vi "Start Process.vi"(0 "Stop / Start Reactor X":refnum<vi>, 1 "System Idle Pressure X":refnum<vi>, 2 "Reactor Number":i32, 3 "Logging Data X":refnum<vi>, 4 "Save File Connection X":refnum<vi>, 5 "Save File JSON Connection X":refnum<vi>, 6 "Header Connection txt Array":refnum<vi>, 7 "Queue Reactor X":refnum<vi>, 8 "Start Time Reactor X":refnum<vi>, 9 "Queue System":refnum<vi>, 10 "Username X":refnum<vi>, 11 "Current Locks":refnum<vi>, 12 "Experimental Details X":refnum<vi>, 13 "System JSON Queue":refnum<vi>, 14 "ALD Sequence for Reactor X":refnum<vi>, 15 "Stop Program":refnum<vi>, 16 "Number of Shared Lines":i32, 17 "Lock Reentrance Rate":u32, 18 "GUID X":refnum<vi>, 19 "Reactor Name":string) -> ()   [LabVIEW 2021]
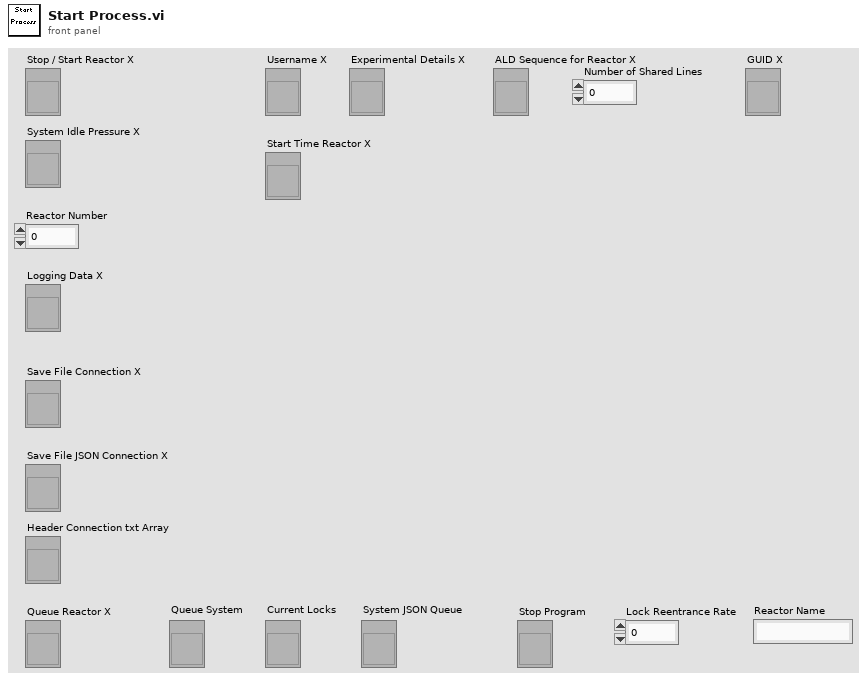
[diagram p1: front panel]
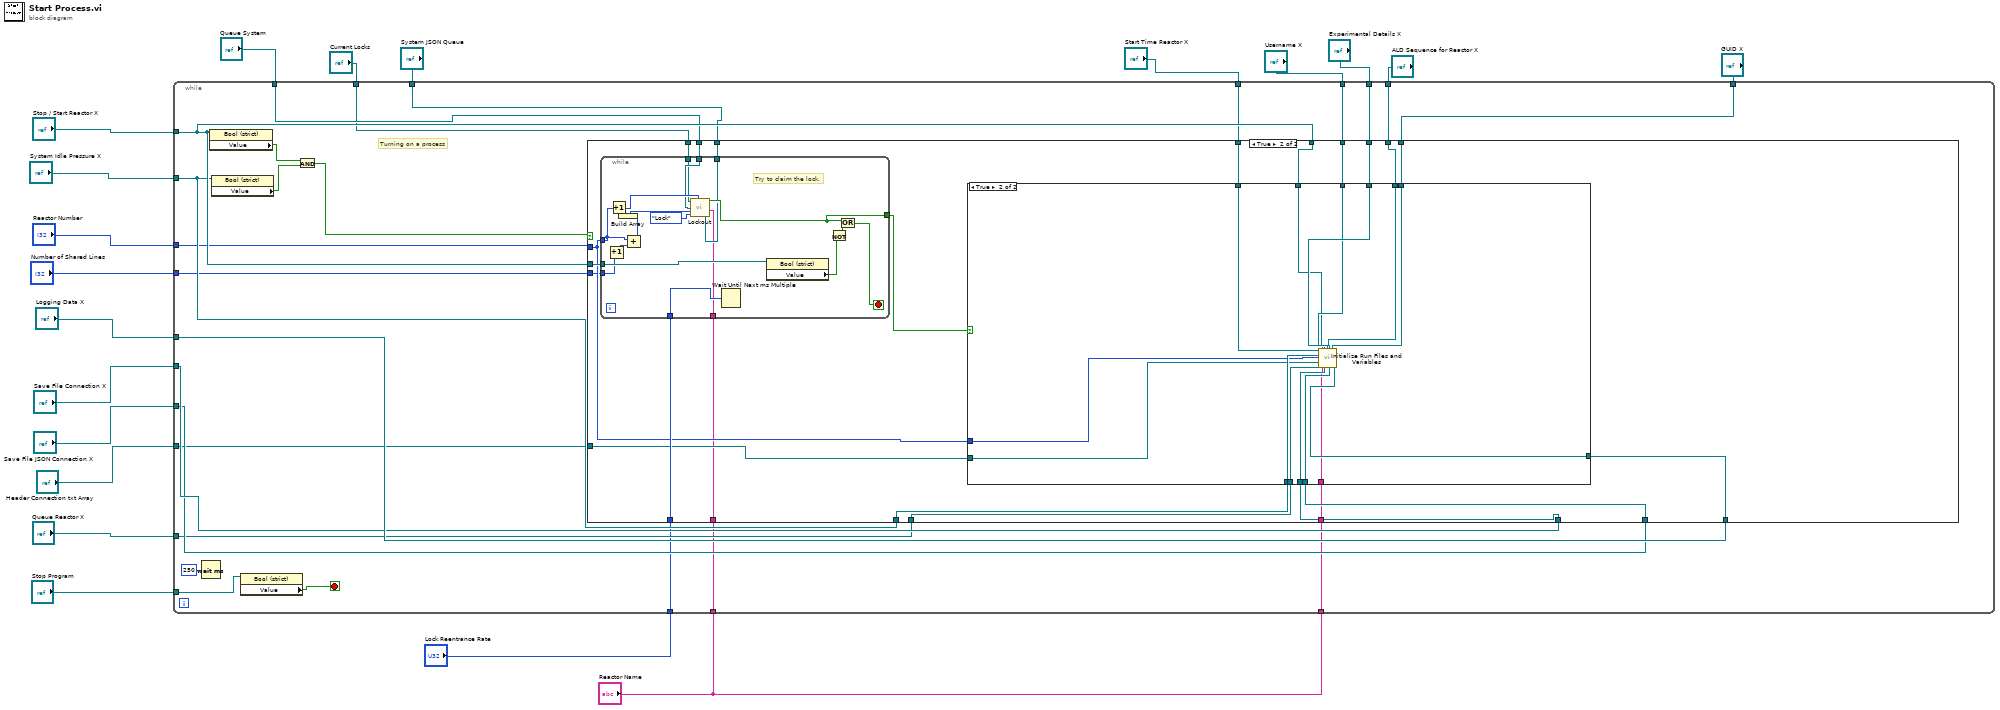
[diagram p0: block diagram]
diagram:
  n1 = while {
    tunnel: "Stop / Start Reactor X" -> [w46]
    tunnel: "System Idle Pressure X" -> [w45]
    tunnel: "Reactor Number" -> [w44]
    tunnel: "Logging Data X" -> [w43]
    tunnel: "Save File Connection X" -> [w41]
    tunnel: "Username X" -> [w40]
    tunnel: "Experimental Details X" -> [w39]
    tunnel: "ALD Sequence for Reactor X" -> [w38]
    tunnel: "Save File JSON Connection X" -> [w37]
    tunnel: "Header Connection txt Array" -> [w36]
    tunnel: "GUID X" -> [w35]
    tunnel: "Queue Reactor X" -> [w34]
    tunnel: "Stop Program" -> [w32]
    tunnel: "Queue System" -> [w31]
    tunnel: "Current Locks" -> [w30]
    tunnel: "System JSON Queue" -> [w29]
    tunnel: "Lock Reentrance Rate" -> [w28]
    tunnel: "Reactor Name" -> [w24]
    tunnel: "Reactor Name" -> [w23]
    tunnel: "Number of Shared Lines" -> [w22]
    tunnel: "Start Time Reactor X" -> [w21]
    stop <- w33 stop-if-true
    # "Turning on a process"
    n2 = Wait (ms)(milliseconds to wait=u32 250 ("millisecond multiple")) -> ()  [unwired: 1 out]
    n3 = property class="Bool (strict)"(reference=w46) -> ("Value"=w26:bool)  [unwired: 1 in, 2 out]
    n4 = property class="Bool (strict)"(reference=w45) -> ("Value"=w27:bool)  [unwired: 1 in, 2 out]
    n5 = property class="Bool (strict)"(reference=w32) -> ("Value"=w33:bool)  [unwired: 1 in, 2 out]
    n6 = And(x=w26, y=w27) -> (x .and. y?=w25:bool)
    n7 = case shown="True" w25 {
      tunnel: w44 -> [_ w57]
      tunnel: w46 -> [_ w68]
      tunnel: w45 -> [_ w58]
      tunnel: w43 -> [_ w52]
      tunnel: w41 -> [_ w54]
      tunnel: w46 -> [_ w59]
      tunnel: w40 -> [_ w60]
      tunnel: w39 -> [_ w61]
      tunnel: w38 -> [_ w62]
      tunnel: w37 -> [_ w53]
      tunnel: w36 -> [_ w56]
      tunnel: w35 -> [_ w63]
      tunnel: w34 -> [_ w55]
      tunnel: w28 -> [_ w67]
      tunnel: w31 -> [_ w66]
      tunnel: w30 -> [_ w65]
      tunnel: w29 -> [_ w64]
      tunnel: w24 -> [_ w50]
      tunnel: w23 -> [_ w49]
      tunnel: w22 -> [_ w48]
      tunnel: w21 -> [_ w47]
      frame False {
        # "If not, do nothing."
      }
      frame True {
        n8 = while {
          tunnel: w57 -> [w85]
          tunnel: [w91] -> w51
          tunnel: w68 -> [w97]
          tunnel: w67 -> [w90]
          tunnel: w66 -> [w89]
          tunnel: w65 -> [w88]
          tunnel: w64 -> [w87]
          tunnel: w49 -> [w86]
          tunnel: w48 -> [w84]
          stop <- w98 stop-if-true
          # "Try to claim the lock."
          n9 = Increment(x=w84) -> (x+1=w83:i32)
          n10 = Increment(x=w85) -> (x+1=w93:i32)
          n11 = Add(x=w85, y=w83) -> (x+y=w95:i32)
          n12 = Build Array(w95) -> (w92:i32[])
          n13 = call "Lockout.vi"("Locks"=w88, "ID"=w93, "Queue System"=w89, "Request Type"=enum16{"Lock", "Release", "Check"}."Lock", "Request Array"=w92, "Reactor Name"=w86, "JSON Queue"=w87) -> ("Response"=w91:bool)  [unwired: 1 out]
          n14 = Wait Until Next ms Multiple(millisecond multiple=w90) -> ()  [unwired: 1 out]
          n15 = property class="Bool (strict)"(reference=w97) -> ("Value"=w99:bool)  [unwired: 1 in, 2 out]
          n16 = Not(x=w99) -> (.not. x?=w96:bool)
          n17 = Or(x=w91, y=w96) -> (x .or. y?=w98:bool)
        }
        n18 = case shown="True" w51 {
          tunnel: w63 -> [_ w82]
          tunnel: w62 -> [_ w81]
          tunnel: w61 -> [_ w80]
          tunnel: w60 -> [_ w79]
          tunnel: w59 -> [_ w78]
          tunnel: w58 -> [_ w77]
          tunnel: w57 -> [_ w76]
          tunnel: w56 -> [_ w75]
          tunnel: w55 -> [_ w74]
          tunnel: w54 -> [_ w73]
          tunnel: w53 -> [_ w72]
          tunnel: w52 -> [_ w71]
          tunnel: w50 -> [_ w70]
          tunnel: w47 -> [_ w69]
          frame False {
          }
          frame True {
            n19 = call "Initialize Run Files and Variables.vi"("Start Time Reactor X"=w69, "System Idle Pressure X"=w77, "Reactor Number"=w76, "Header Connection txt Array"=w75, "Queue Reactor X"=w74, "Stop / Start Reactor X"=w78, "Reactor Name"=w70, "Username X"=w79, "Save File Connection X"=w73, "Experimental Details X"=w80, "ALD Sequence for Reactor X"=w81, "Save File JSON Connection X"=w72, "GUID X"=w82, "Logging Data X"=w71) -> ()  [unwired: 14 in]
          }
        }
      }
    }
  }
